vi "Material Theme Editor.vi"() -> ()   [LabVIEW 2021]
doc: "Convert existing material3 json files exported from Google to be used with TSC Material application VIs.\n\n<b>Code Developed By:</b>\nDaniel Coons\nTechnology Service Corporation\nwww.tsc.com/atcs"
uses:
  Material Theme/Material Theme.lvclass
  <vilib>/Utility/traverseref.llb/TRef TravTarget.ctl
  _theme-editor/Theme Config/Theme Config.lvclass/Theme Config.ctl
  _Material Theme SubVIs/material theme.ctl
  _Material Theme SubVIs/material json scheme.ctl
  _Material Theme SubVIs/material json palette.ctl
  Material-Scheme/Material-Scheme.lvclass/Material-Scheme.ctl
  8aff6bdd-0f42-4725-a4f4-6aecb987c99b.vi
  _theme-editor/Theme Config/Set theme path.vi
  _theme-editor/Theme Config/Set Theme Mode.vi
  Material-Scheme/data member access/get surface.vi
  Material-Scheme/data member access/Read name.vi
  _theme-editor/Theme Config/Get theme path.vi
  _theme-editor/Theme Config/Get Theme Mode.vi
  <vilib>/JDP Science/JSONtext/JSON text to Variant.vi
  _theme-editor/Theme Config/Save Configuration.vi
  Material-Scheme/View-User Colors.vi
  Material-Scheme/Material-Scheme.lvclass
  <vilib>/JDP Science/JSONtext/LVClass Serializer/JSONtext LVClass Serializer.lvclass
  Material-Palette/Material-Palette.lvclass
  user32.dll
  <vilib>/Utility/traverseref.llb/VI Scripting - Traverse.lvlib
  _theme-editor/Theme Config/Theme Config.lvclass
panel:
  in  "palette":bool
  in  "File Interaction":enum32{"convert--buton", "load--buton"}(radio)
  in  "tabs":enum32{"color", "palette", "json", "buttons"}(radio)
  in  "preview":bool
  in  "close":bool
  out "header":bool
  in  "save":bool
  in  "Theme Mode":u16(ring) items=["Light Theme", "Light Medium Contrast", "Light High Contrast", "Dark Theme", "Dark Medium Contrast", "Dark High Constrast"]
  in  "Tab Control":T1(tab)
  out "material JSON output":string
  in  "Color Level":u16(ring) items=["Primary", "Secondary", "Tertiary", "Error", "Primary Fixed", "Secondary Fixed", "Tertiary Fixed"]
  in  "Tab Control file":enum32{"convert", "load"}(tab)
  in  "json file path":path
  in  "LabVIEW material theme":path
  # "Convert a JSON M3 theme file from Google and \nuse the TSC Material Theme in a VI"
  # "Can be generated through Figma or at:   https://material-foundation.github.io/material-theme-builder/<Material Website>"
  # "Load a TSC Material Theme LabVIEW file to see modes\nand palette colors."
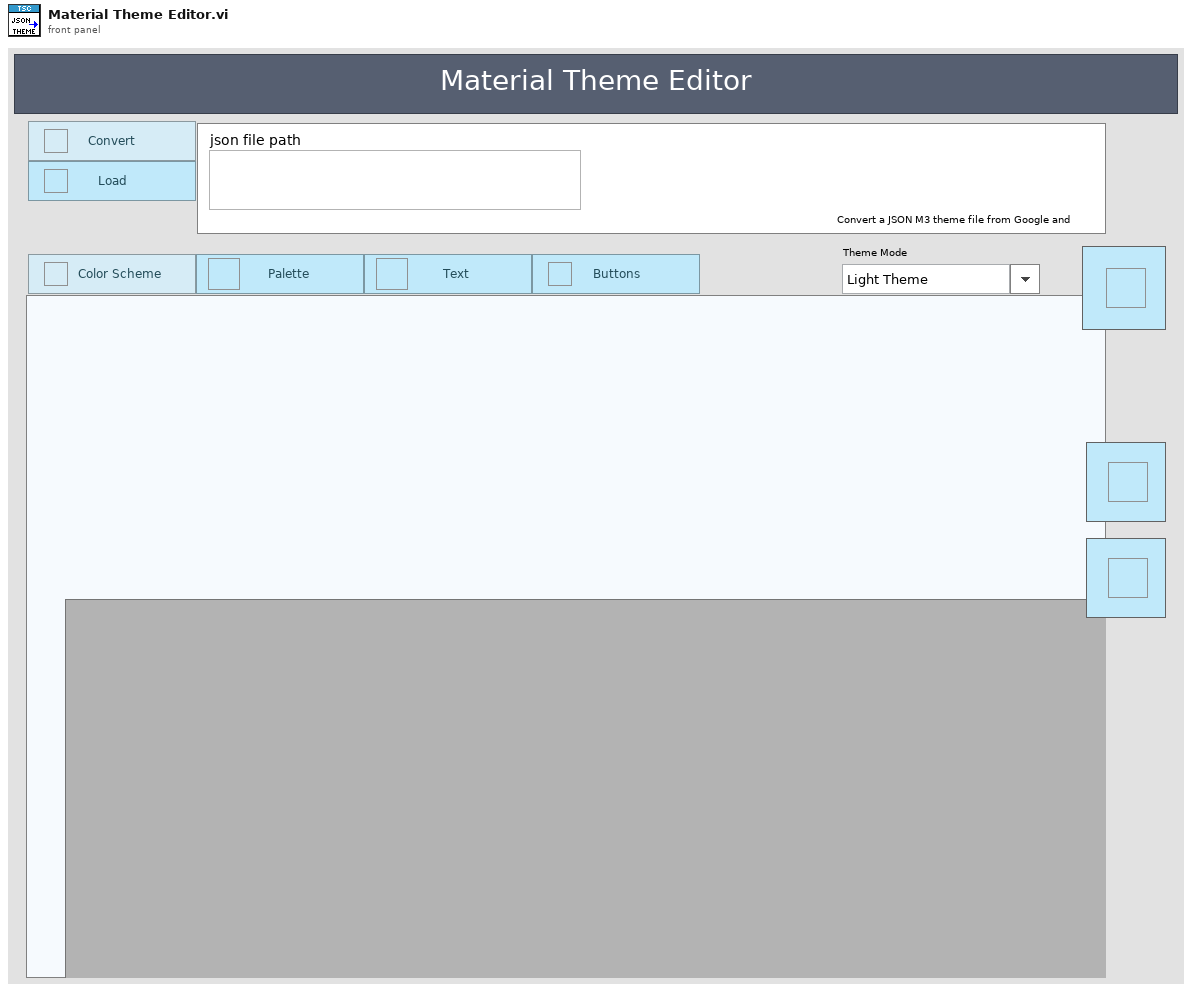
[diagram p1: front panel]
types:
  T1 = enum32{"Color Scheme", "Palette Variations", "JSON String", "buttons"}
  T2 = typedef "TRef TravTarget.ctl" = enum16{"FP", "BD", "Other"}
  T3 = typedef "material theme.ctl" = cluster{"description":string, "seed":string, "coreColors":cluster{"primary":string, "secondary":string, "tertiary":string, "error":string}, "schemes":cluster{"light":T4, "light-medium-contrast":T4, "light-high-contrast":T4, "dark":T4, "dark-medium-contrast":T4, "dark-high-contrast":T4}, "palettes":cluster{"primary":T5, "secondary":T5, "tertiary":T5, "neutral":T5, "neutral-variant":T5}}
  T4 = typedef "material json scheme.ctl" = cluster{"primary":string, "surfaceTint":string, "onPrimary":string, "primaryContainer":string, "onPrimaryContainer":string, "secondary":string, "onSecondary":string, "secondaryContainer":string, "onSecondaryContainer":string, "tertiary":string, "onTertiary":string, "tertiaryContainer":string, "onTertiaryContainer":string, "error":string, "onError":string, "errorContainer":string, "onErrorContainer":string, "background":string, "onBackground":string, "surface":string, "onSurface":string, "surfaceVariant":string, "onSurfaceVariant":string, "outline":string, "outlineVariant":string, "shadow":string, "scrim":string, "inverseSurface":string, "inverseOnSurface":string, "inversePrimary":string, "primaryFixed":string, "onPrimaryFixed":string, "primaryFixedDim":string, "onPrimaryFixedVariant":string, "secondaryFixed":string, "onSecondaryFixed":string, "secondaryFixedDim":string, "onSecondaryFixedVariant":string, "tertiaryFixed":string, "onTertiaryFixed":string, "tertiaryFixedDim":string, "onTertiaryFixedVariant":string, "surfaceDim":string, "surfaceBright":string, "surfaceContainerLowest":string, "surfaceContainerLow":string, "surfaceContainer":string, "surfaceContainerHigh":string, "surfaceContainerHighest":string}
  T5 = typedef "material json palette.ctl" = cluster{"0":string, "5":string, "10":string, "15":string, "20":string, "25":string, "30":string, "35":string, "40":string, "50":string, "60":string, "70":string, "80":string, "90":string, "95":string, "98":string, "99":string, "100":string}
  T6 = enum16{"open", "replace", "create", "open or create", "replace or create", "replace or create with confirmation"}
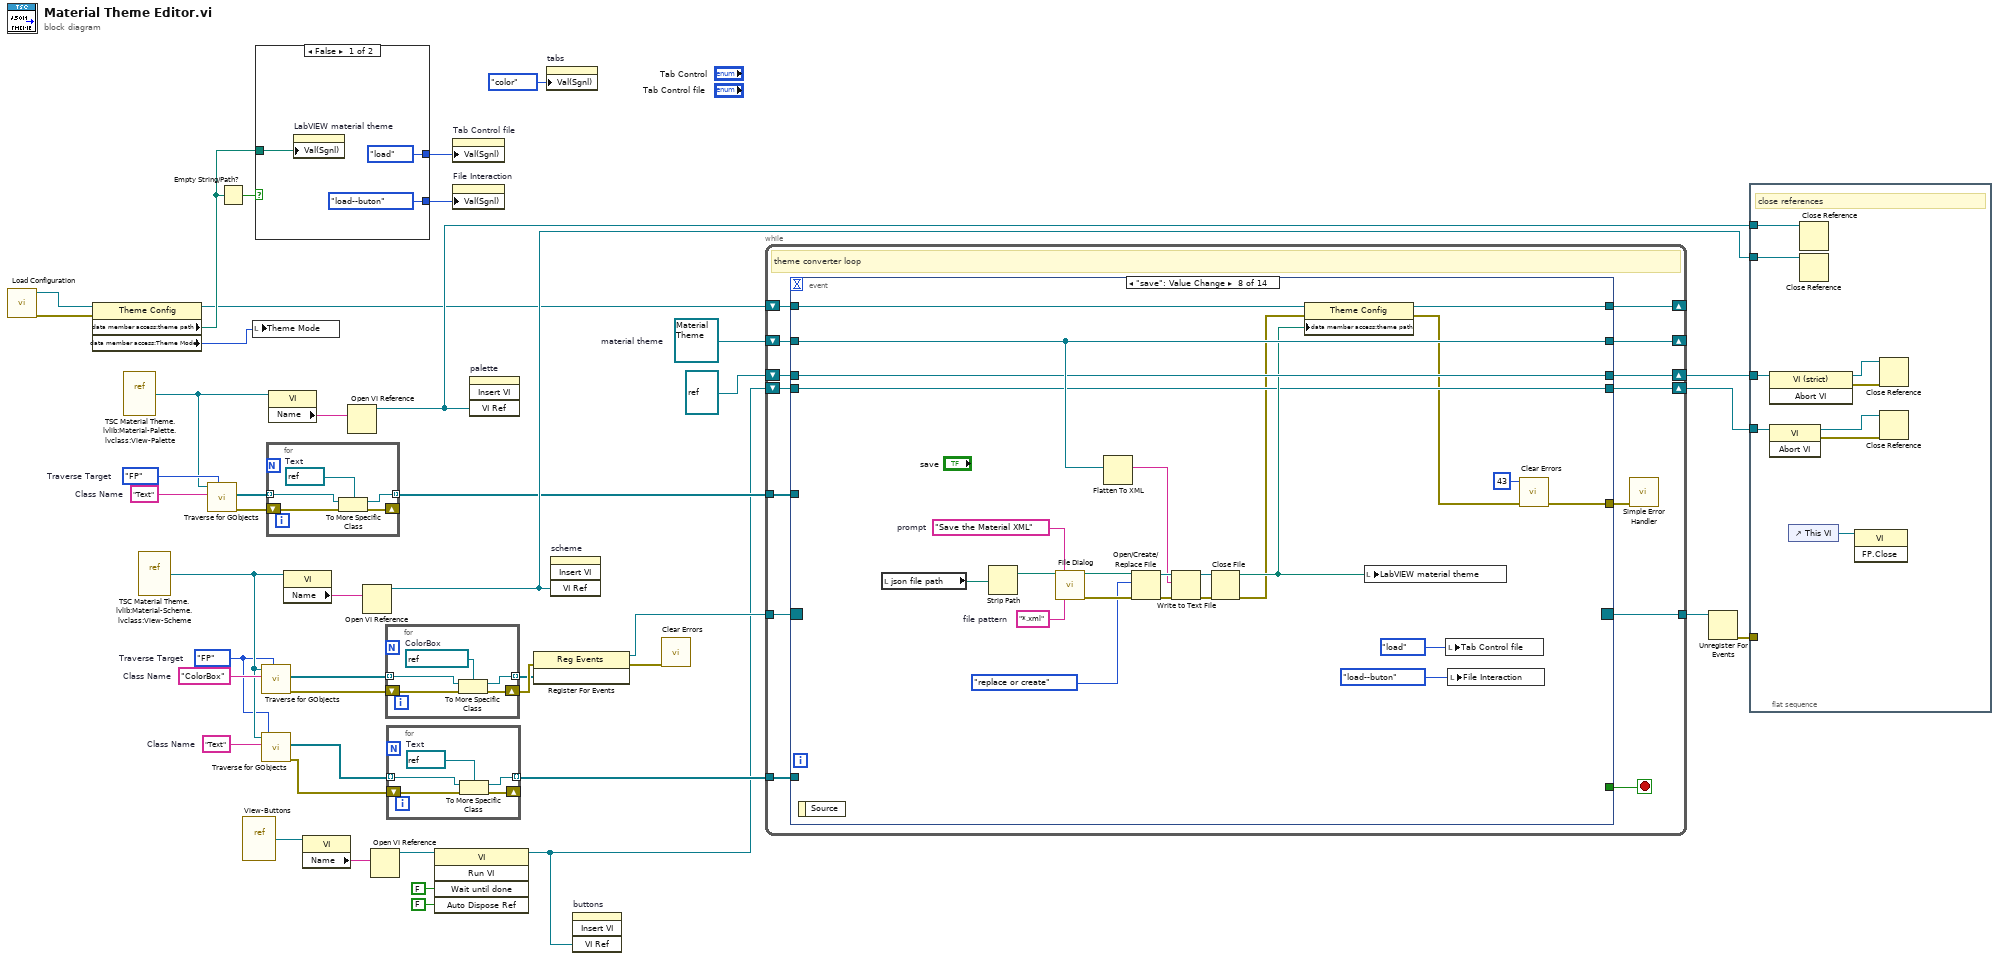
[diagram p0: block diagram]
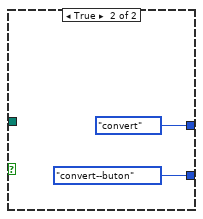
[diagram p2: hidden frame]
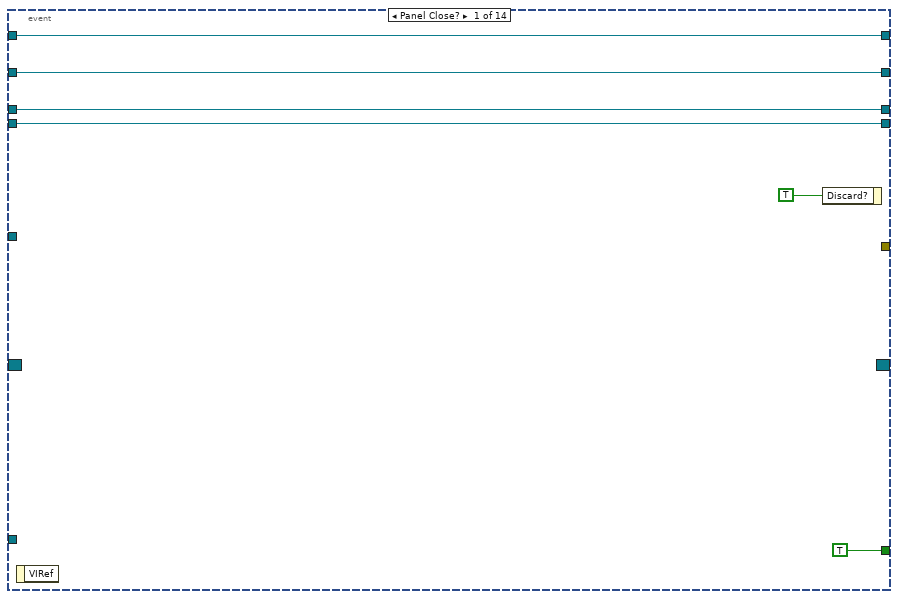
[diagram p3: hidden frame]
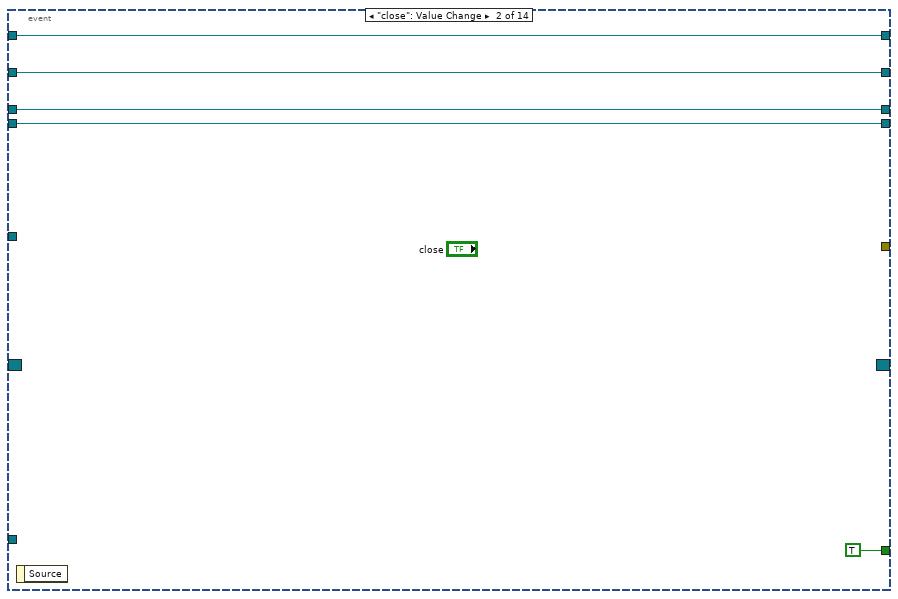
[diagram p4: hidden frame]
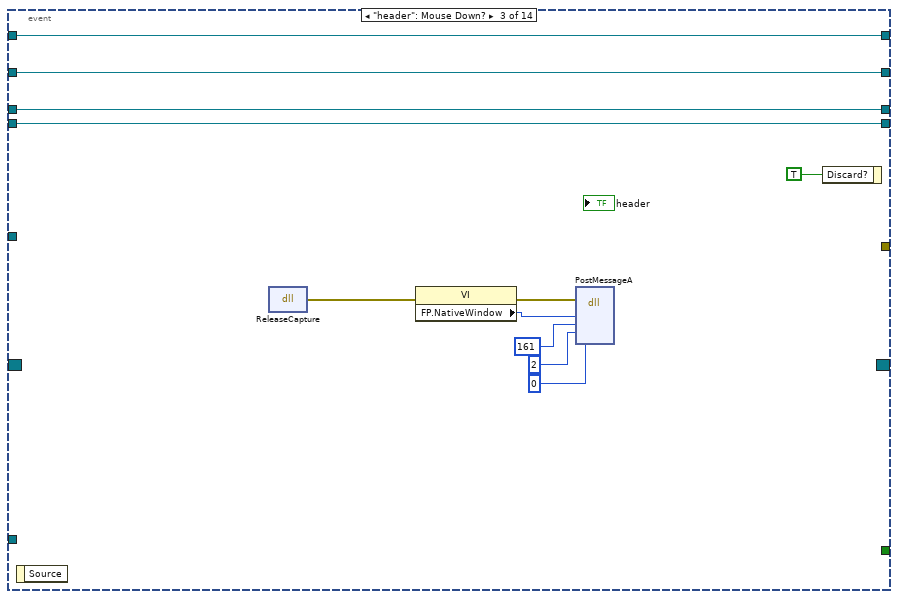
[diagram p5: hidden frame]
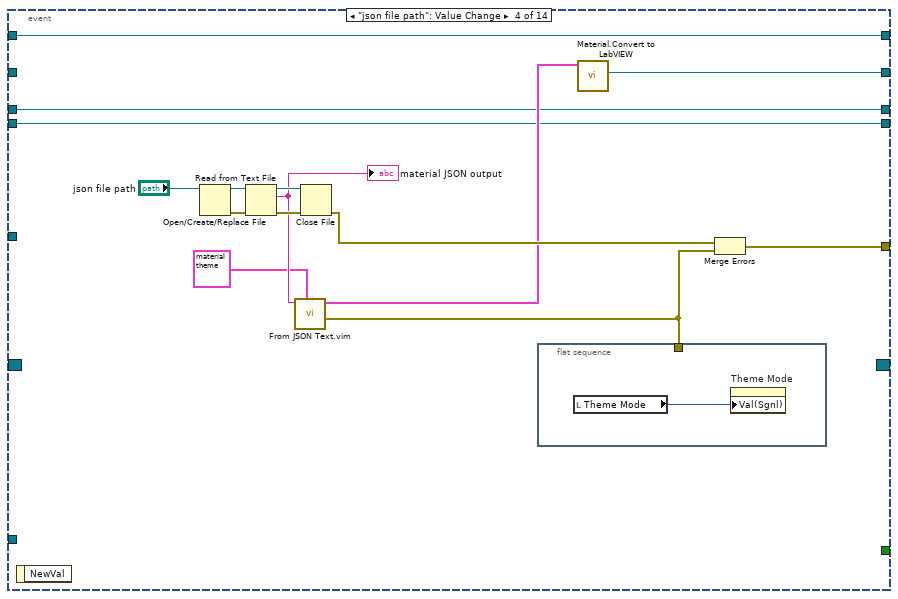
[diagram p6: hidden frame]
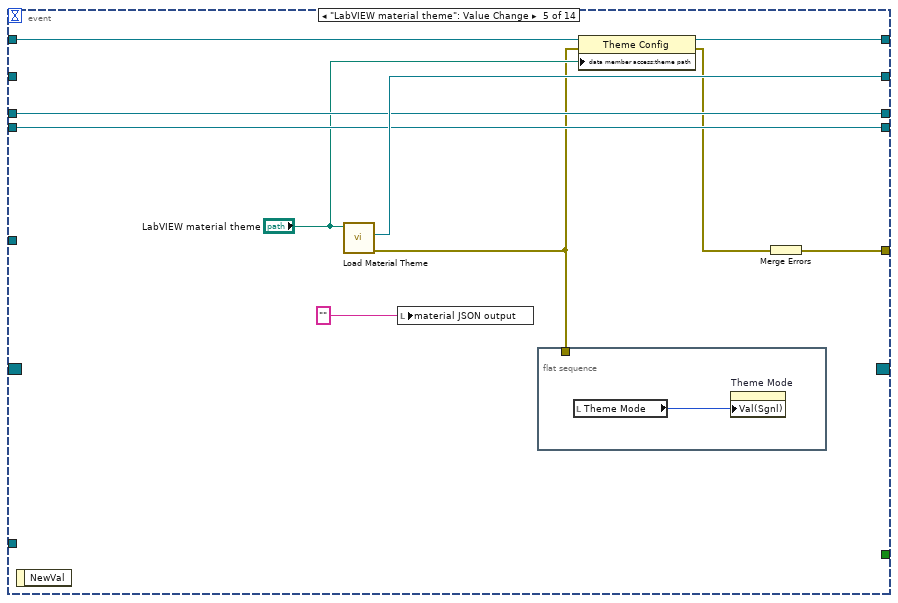
[diagram p7: hidden frame]
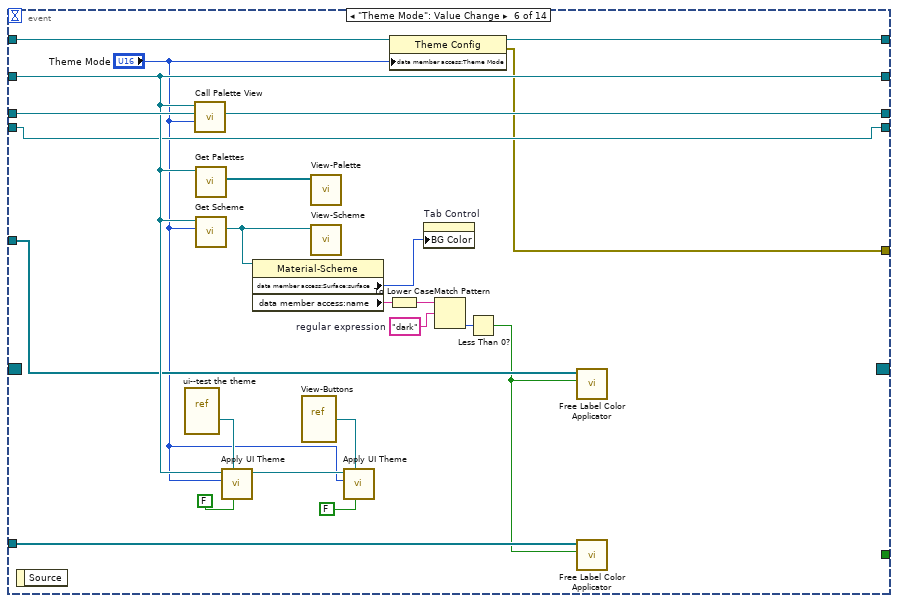
[diagram p8: hidden frame]
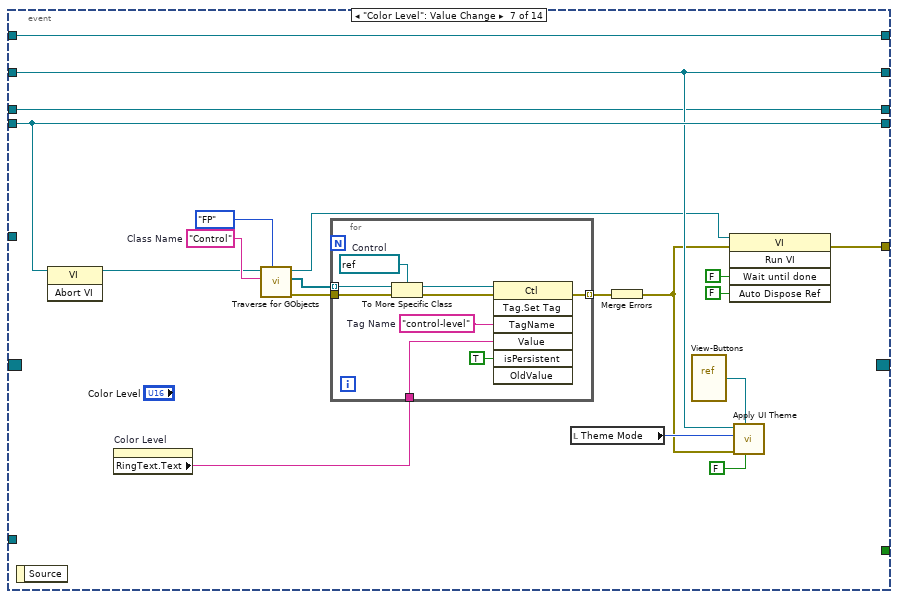
[diagram p9: hidden frame]
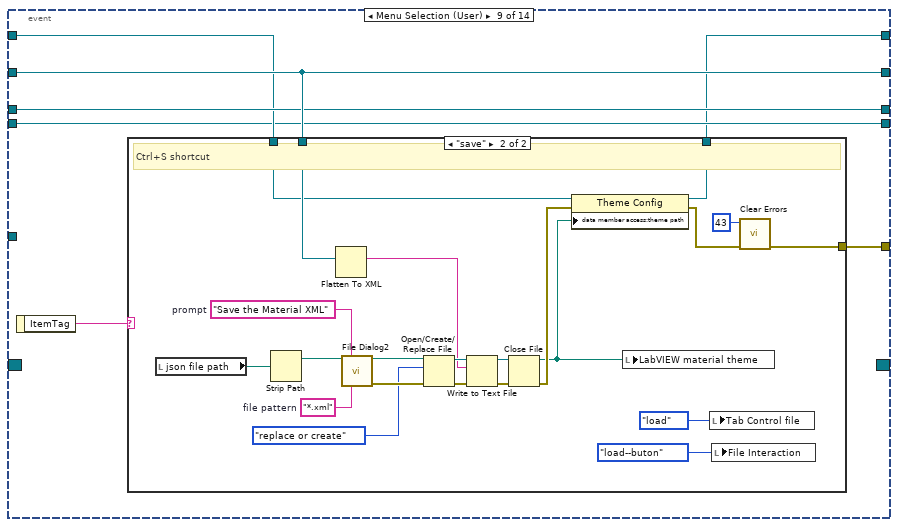
[diagram p10: hidden frame]
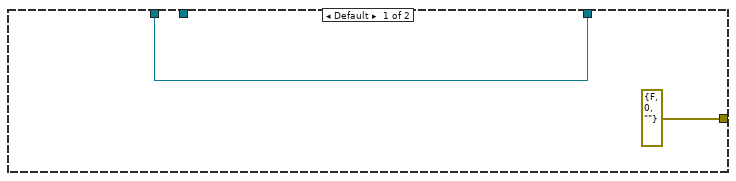
[diagram p11: hidden frame]
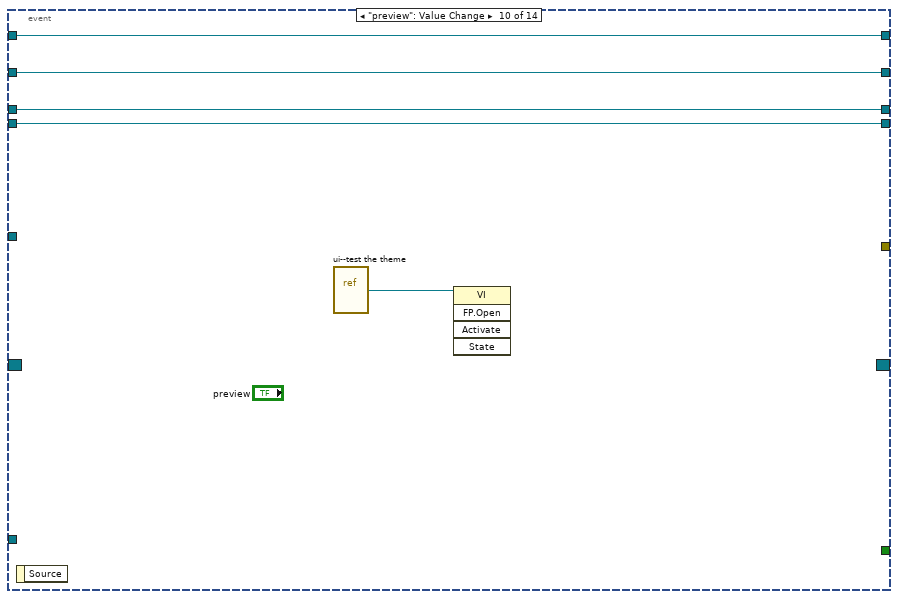
[diagram p12: hidden frame]
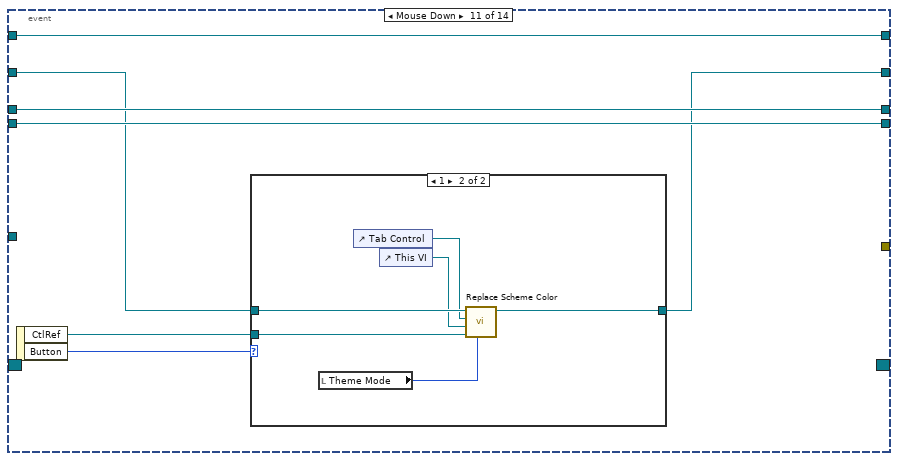
[diagram p13: hidden frame]
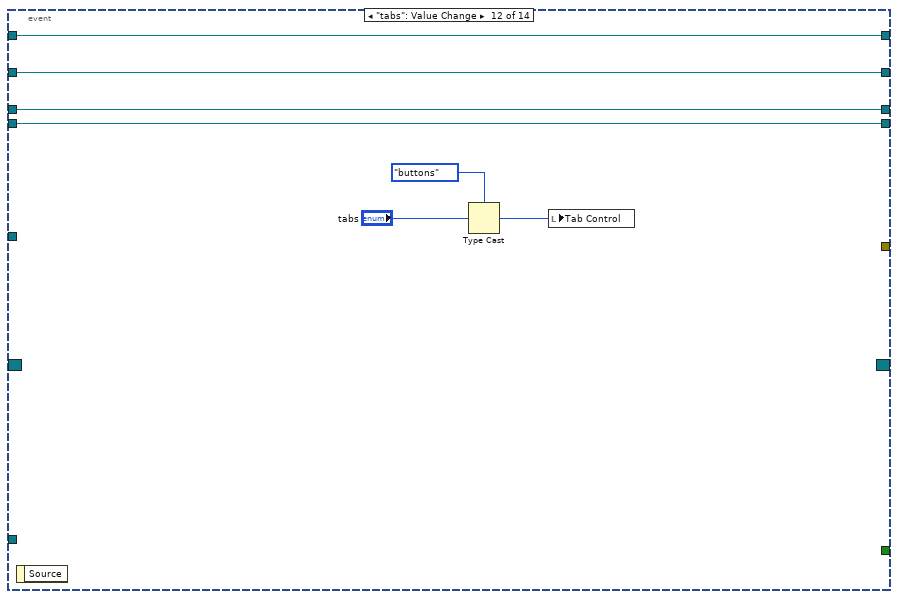
[diagram p15: hidden frame]
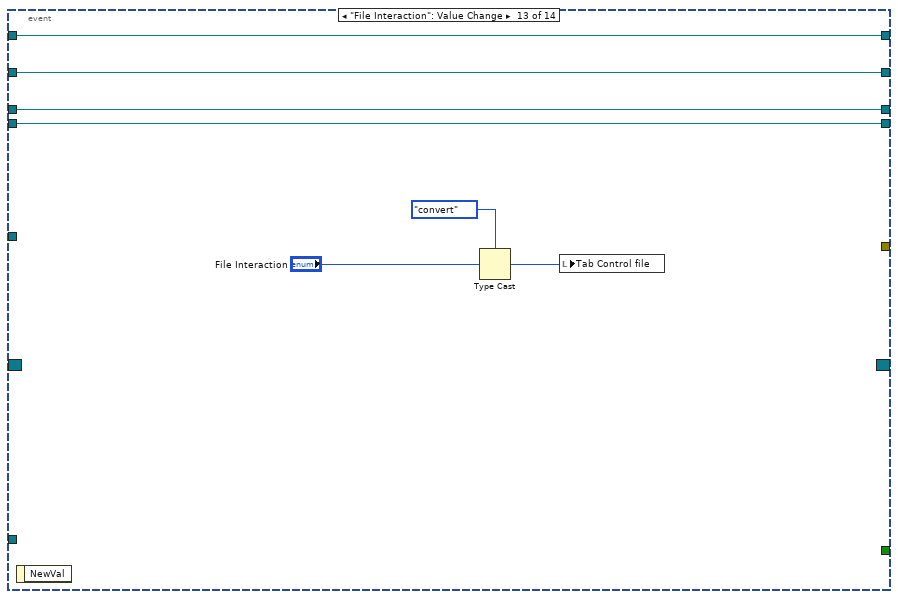
[diagram p16: hidden frame]
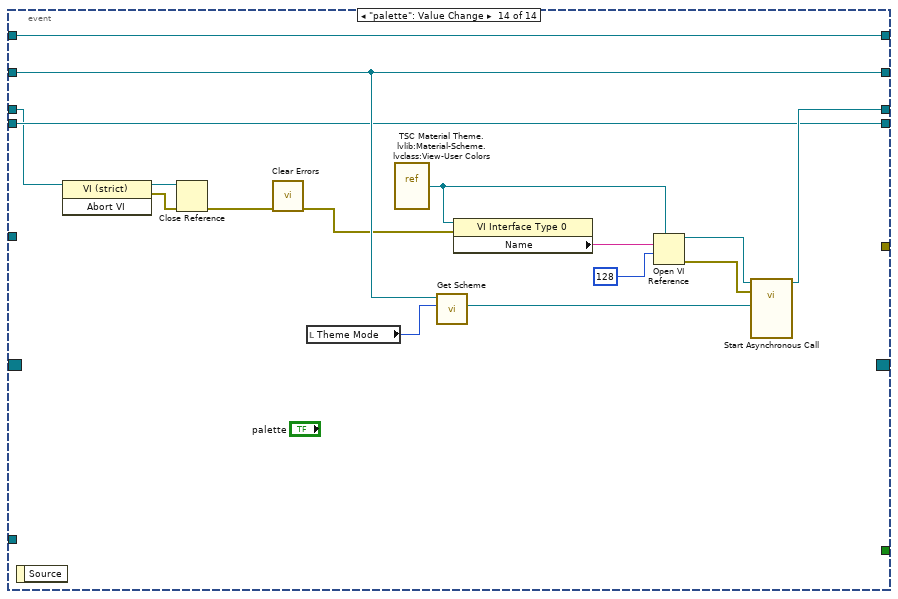
[diagram p17: hidden frame]
diagram:
  w24 = "Text"  # Class Name
  w27 = "Text"  # Class Name
  w28 = TRef_TravTarget."FP"  # Traverse Target
  w30 = refnum<class "Material Theme.lvclass"> refnum  # material theme
  w36 = "ColorBox"  # Class Name
  w22 = TRef_TravTarget."FP"  # Traverse Target
  n1 = call "Load Configuration.vi"() -> ("error out"=w10:errorcluster, "Theme Config out"=w9:refnum<class "Theme Config.lvclass">)  [unwired: 10 in]
  n2 = property class="Theme Config"(reference=w9, error in=w10) -> (reference out=w6:refnum<class "Theme Config.lvclass">, "data member access:theme path"=w8:path, "data member access:Theme Mode"=w3:u16)  [unwired: 1 out]
  n3 = vi-ref "TSC Material Theme.lvlib:Material-Palette.lvclass:View-Palette.vi"() -> (w7:refnum<vi>)
  n4 = vi-ref "TSC Material Theme.lvlib:Material-Scheme.lvclass:View-Scheme.vi"() -> (w23:refnum<vi>)
  n5 = call <vilib>:"Traverse for GObjects.vi"("Traverse Target"=w28, "Class Name"=w27, "VI Refnum"=w7) -> ("error out"=w41:errorcluster, "References"=w26:refnum<vi>[])  [unwired: 5 in, 2 out]
  n6 = Empty String/Path?(string/path=w8) -> (empty?=w29:bool)
  n7 = vi-ref "View-Buttons.vi"() -> (w17:refnum<vi>)
  n8 = local write "Theme Mode"(w3) -> ()
  n9 = case shown="False" w29 {
    tunnel: w8 -> [w47 _]
    tunnel: [enum32{"convert", "load"}."load" ("Value (Signaling)") enum32{"convert", "load"}."convert" ("Value (Signaling)")] -> w2
    tunnel: [enum32{"convert--buton", "load--buton"}."load--buton" ("Value (Signaling)") enum32{"convert--buton", "load--buton"}."convert--buton" ("Value (Signaling)")] -> w1
    frame False {
      n10 = property on="LabVIEW material theme" class="Path"("Val(Sgnl)"=w47) -> ()  [unwired: 2 in, 2 out]
    }
    frame True {
    }
  }
  n11 = call <vilib>:"Traverse for GObjects.vi"("Traverse Target"=w22, "Class Name"=w36, "VI Refnum"=w23) -> ("error out"=w44:errorcluster, "References"=w34:refnum<vi>[])  [unwired: 5 in, 2 out]
  n12 = call <vilib>:"Traverse for GObjects.vi"("Traverse Target"=w22, "Class Name"=w24, "VI Refnum"=w23) -> ("error out"=w40:errorcluster, "References"=w21:refnum<vi>[])  [unwired: 5 in, 2 out]
  n13 = for {
    tunnel: w26 -> [w51] mode=indexing
    shift-right: [w53] -> _
    shift-left: w41 -> [w54]
    tunnel: [w50] -> w25 mode=indexing
    w52 = refnum<vi> refnum  # Text
    n14 = To More Specific Class(target class=w52, reference=w51, error in=w54) -> (specific class reference=w50:refnum<vi>, error out=w53:errorcluster)
  }
  n15 = property class="VI"(reference=w7) -> ("Name"=w39:string)  [unwired: 1 in, 2 out]
  n16 = property class="VI"(reference=w23) -> ("Name"=w38:string)  [unwired: 1 in, 2 out]
  n17 = property class="VI"(reference=w17) -> ("Name"=w16:string)  [unwired: 1 in, 2 out]
  n18 = Open VI Reference(vi path=w39) -> (vi reference=w37:refnum<vi>)  [unwired: 5 in, 1 out]
  n19 = Open VI Reference(vi path=w38) -> (vi reference=w33:refnum<vi>)  [unwired: 5 in, 1 out]
  n20 = Open VI Reference(vi path=w16) -> (vi reference=w18:refnum<vi>)  [unwired: 5 in, 1 out]
  n21 = for {
    tunnel: w34 -> [w56] mode=indexing
    shift-right: [w58] -> w43
    shift-left: w44 -> [w59]
    tunnel: [w55] -> w32 mode=indexing
    w57 = refnum<vi> refnum  # ColorBox
    n22 = To More Specific Class(target class=w57, reference=w56, error in=w59) -> (specific class reference=w55:refnum<vi>, error out=w58:errorcluster)
  }
  n23 = for {
    tunnel: w21 -> [w61] mode=indexing
    shift-right: [w63] -> _
    shift-left: w40 -> [w64]
    tunnel: [w60] -> w20 mode=indexing
    w62 = refnum<vi> refnum  # Text
    n24 = To More Specific Class(target class=w62, reference=w61, error in=w64) -> (specific class reference=w60:refnum<vi>, error out=w63:errorcluster)
  }
  n25 = invoke class="VI" method="Run VI"(reference=w18, "Wait until done"=FALSE ("Wait Until Done"), "Auto Dispose Ref"=FALSE ("Auto Dispose Reference")) -> (reference out=w13:refnum<vi>)  [unwired: 2 in, 4 out]
  n26 = property on="Tab Control file" class="TabCtl (strict)"("Val(Sgnl)"=w2) -> ()  [unwired: 2 in, 2 out]
  n27 = property on="File Interaction" class="RadioBtnsControl (strict)"("Val(Sgnl)"=w1) -> ()  [unwired: 2 in, 2 out]
  n28 = invoke on="palette" class="SubPnl" method="Insert VI"("VI Ref"=w37) -> ()  [unwired: 3 in, 4 out]
  n29 = register-events(error in=w43, w32) -> (reference out=w35:refnum<event-registration>, error out=w42:errorcluster)  [unwired: 1 in]
  n30 = property on="tabs" class="RadioBtnsControl (strict)"("Val(Sgnl)"=enum32{"color", "palette", "json", "buttons"}."color" ("Value (Signaling)")) -> ()  [unwired: 2 in, 2 out]
  n31 = invoke on="scheme" class="SubPnl" method="Insert VI"("VI Ref"=w33) -> ()  [unwired: 3 in, 4 out]
  n32 = invoke on="buttons" class="SubPnl" method="Insert VI"("VI Ref"=w13) -> ()  [unwired: 3 in, 4 out]
  n33 = call <vilib>:"Clear Errors.vi"("error in (no error)"=w42) -> ()  [unwired: 5 in, 2 out]
  n34 = while {
    shift-right: [w76] -> _
    shift-left: w30 -> [w75]
    tunnel: w35 -> [w74]
    tunnel: [w73] -> w31
    tunnel: w25 -> [w72]
    tunnel: w20 -> [w71]
    shift-right: [w69] -> w12
    shift-left: refnum<vi> refnum -> [w68]
    shift-right: [w66] -> _
    shift-left: w6 -> [w67]
    shift-right: [w65] -> w4
    shift-left: w13 -> [w70]
    stop <- w77 stop-if-true
    # "theme converter loop"
    n35 = event shown="[7] \"save\": Value Change" {
      selector: w74 -> [_ _ _ _ _ _ _ _ _ _ _ _ _ _]
      dyn-events: [_ _ _ _ _ _ _ _ _ _ _ _ _ _] -> w73
      timeout: _ -> [_ _ _ _ _ _ _ _ _ _ _ _ _ _]
      tunnel: [TRUE TRUE _ _ _ _ _ _ _ _ _ _ _ _] -> w77
      tunnel: [w82 w89 w93 w108 w125 w137 w156 w196 w208 w238 w239 w259 w263 w282] -> w76
      tunnel: w75 -> [w82 w89 w93 _ _ w137 w156 w196 w208 w238 w240 w259 w263 w282]
      tunnel: [_ _ _ w112 w126 w128 w162 w179 w209 _ _ _ _ _] -> w78
      tunnel: w72 -> [_ _ _ _ _ w132 _ _ _ _ _ _ _ _]
      tunnel: w71 -> [_ _ _ _ _ w141 _ _ _ _ _ _ _ _]
      tunnel: w70 -> [w79 w85 w90 w101 w121 w133 w167 w182 w204 w234 w242 w253 w260 w272]
      tunnel: [w81 w87 w92 w103 w123 w136 w152 w188 w206 w236 w244 w255 w262 w274] -> w69
      tunnel: w68 -> [w81 w87 w92 w103 w123 w138 w152 w188 w206 w236 w244 w255 w262 w269]
      tunnel: w67 -> [w80 w86 w91 w102 w122 w134 w151 w185 w205 w235 w243 w254 w261 w273]
      tunnel: [w80 w86 w91 w102 w120 w130 w151 w184 w203 w235 w243 w254 w261 w273] -> w66
      tunnel: [w79 w85 w90 w101 w121 w133 w167 w182 w204 w234 w242 w253 w260 w272] -> w65
      event Panel Close? {
        n36 = event-data() -> ()  [unwired: 1 in, 1 out]
        n37 = event-data("Discard?"=TRUE) -> ()  [unwired: 1 in, 1 out]
      }
      event "close": Value Change {
        n38 = event-data() -> ()  [unwired: 1 in, 1 out]
      }
      event "header": Mouse Down? {
        n39 = event-data() -> ()  [unwired: 1 in, 1 out]
        n40 = dll-call lib="user32.dll" fn="ReleaseCapture"() -> (error out=w100:errorcluster)  [unwired: 4 in, 1 out]
        n41 = property class="VI"(error in=w100) -> (error out=w99:errorcluster, "FP.NativeWindow"=w94:u64)  [unwired: 1 in, 1 out]
        n42 = dll-call lib="user32.dll" fn="PostMessageA"(error in=w99, "hWnd"=w94, "Msg"=161, "wParam"=2, "lParam"=0) -> ()  [unwired: 7 in, 2 out]
        n43 = event-data("Discard?"=TRUE) -> ()  [unwired: 1 in, 1 out]
      }
      event "json file path": Value Change {
        n44 = event-data() -> ()  [unwired: 1 in, 1 out]
        n45 = Open/Create/Replace File(file path (use dialog)="json file path") -> (refnum out=w109:refnum<file>, error out=w114:errorcluster)  [unwired: 5 in, 1 out]
        n46 = Read from Text File(file (use dialog)=w109, error in=w114) -> (refnum out=w110:refnum<file>, text=w107:string, error out=w115:errorcluster)  [unwired: 2 in, 1 out]
        "material JSON output" <- w107
        n47 = call "From JSON Text.vim"("Data Type and Default Value"=T3 {"description"="", "seed"="", "coreColors"={"primary"="", "secondary"="", "tertiary"="", "error"=""}, "schemes"={"light"={"primary"="", "surfaceTint"="", "onPrimary"="", "primaryContainer"="0", "onPrimaryContainer"="0", "secondary"="0", "onSecondary"="0", "secondaryContainer"="0", "onSecondaryContainer"="0", "tertiary"="0", "onTertiary"="0", "tertiaryContainer"="0", "onTertiaryContainer"="0", "error"="0", "onError"="0", "errorContainer"="0", "onErrorContainer"="0", "background"="0", "onBackground"="0", "surface"="0", "onSurface"="0", "surfaceVariant"="0", "onSurfaceVariant"="0", "outline"="0", "outlineVariant"="0", "shadow"="0", "scrim"="0", "inverseSurface"="0", "inverseOnSurface"="0", "inversePrimary"="", "primaryFixed"="0", "onPrimaryFixed"="0", "primaryFixedDim"="0", "onPrimaryFixedVariant"="0", "secondaryFixed"="0", "onSecondaryFixed"="0", "secondaryFixedDim"="0", "onSecondaryFixedVariant"="0", "tertiaryFixed"="0", "onTertiaryFixed"="0", "tertiaryFixedDim"="0", "onTertiaryFixedVariant"="0", "surfaceDim"="0", "surfaceBright"="0", "surfaceContainerLowest"="0", "surfaceContainerLow"="0", "surfaceContainer"="0", "surfaceContainerHigh"="0", "surfaceContainerHighest"="0"}, "light-medium-contrast"={"primary"="", "surfaceTint"="", "onPrimary"="", "primaryContainer"="0", "onPrimaryContainer"="0", "secondary"="0", "onSecondary"="0", "secondaryContainer"="0", "onSecondaryContainer"="0", "tertiary"="0", "onTertiary"="0", "tertiaryContainer"="0", "onTertiaryContainer"="0", "error"="0", "onError"="0", "errorContainer"="0", "onErrorContainer"="0", "background"="0", "onBackground"="0", "surface"="0", "onSurface"="0", "surfaceVariant"="0", "onSurfaceVariant"="0", "outline"="0", "outlineVariant"="0", "shadow"="0", "scrim"="0", "inverseSurface"="0", "inverseOnSurface"="0", "inversePrimary"="", "primaryFixed"="0", "onPrimaryFixed"="0", "primaryFixedDim"="0", "onPrimaryFixedVariant"="0", "secondaryFixed"="0", "onSecondaryFixed"="0", "secondaryFixedDim"="0", "onSecondaryFixedVariant"="0", "tertiaryFixed"="0", "onTertiaryFixed"="0", "tertiaryFixedDim"="0", "onTertiaryFixedVariant"="0", "surfaceDim"="0", "surfaceBright"="0", "surfaceContainerLowest"="0", "surfaceContainerLow"="0", "surfaceContainer"="0", "surfaceContainerHigh"="0", "surfaceContainerHighest"="0"}, "light-high-contrast"={"primary"="", "surfaceTint"="", "onPrimary"="", "primaryContainer"="0", "onPrimaryContainer"="0", "secondary"="0", "onSecondary"="0", "secondaryContainer"="0", "onSecondaryContainer"="0", "tertiary"="0", "onTertiary"="0", "tertiaryContainer"="0", "onTertiaryContainer"="0", "error"="0", "onError"="0", "errorContainer"="0", "onErrorContainer"="0", "background"="0", "onBackground"="0", "surface"="0", "onSurface"="0", "surfaceVariant"="0", "onSurfaceVariant"="0", "outline"="0", "outlineVariant"="0", "shadow"="0", "scrim"="0", "inverseSurface"="0", "inverseOnSurface"="0", "inversePrimary"="", "primaryFixed"="0", "onPrimaryFixed"="0", "primaryFixedDim"="0", "onPrimaryFixedVariant"="0", "secondaryFixed"="0", "onSecondaryFixed"="0", "secondaryFixedDim"="0", "onSecondaryFixedVariant"="0", "tertiaryFixed"="0", "onTertiaryFixed"="0", "tertiaryFixedDim"="0", "onTertiaryFixedVariant"="0", "surfaceDim"="0", "surfaceBright"="0", "surfaceContainerLowest"="0", "surfaceContainerLow"="0", "surfaceContainer"="0", "surfaceContainerHigh"="0", "surfaceContainerHighest"="0"}, "dark"={"primary"="", "surfaceTint"="", "onPrimary"="", "primaryContainer"="0", "onPrimaryContainer"="0", "secondary"="0", "onSecondary"="0", "secondaryContainer"="0", "onSecondaryContainer"="0", "tertiary"="0", "onTertiary"="0", "tertiaryContainer"="0", "onTertiaryContainer"="0", "error"="0", "onError"="0", "errorContainer"="0", "onErrorContainer"="0", "background"="0", "onBackground"="0", "surface"="0", "onSurface"="0", "surfaceVariant"="0", "onSurfaceVariant"="0", "outline"="0", "outlineVariant"="0", "shadow"="0", "scrim"="0", "inverseSurface"="0", "inverseOnSurface"="0", "inversePrimary"="", "primaryFixed"="0", "onPrimaryFixed"="0", "primaryFixedDim"="0", "onPrimaryFixedVariant"="0", "secondaryFixed"="0", "onSecondaryFixed"="0", "secondaryFixedDim"="0", "onSecondaryFixedVariant"="0", "tertiaryFixed"="0", "onTertiaryFixed"="0", "tertiaryFixedDim"="0", "onTertiaryFixedVariant"="0", "surfaceDim"="0", "surfaceBright"="0", "surfaceContainerLowest"="0", "surfaceContainerLow"="0", "surfaceContainer"="0", "surfaceContainerHigh"="0", "surfaceContainerHighest"="0"}, "dark-medium-contrast"={"primary"="", "surfaceTint"="", "onPrimary"="", "primaryContainer"="0", "onPrimaryContainer"="0", "secondary"="0", "onSecondary"="0", "secondaryContainer"="0", "onSecondaryContainer"="0", "tertiary"="0", "onTertiary"="0", "tertiaryContainer"="0", "onTertiaryContainer"="0", "error"="0", "onError"="0", "errorContainer"="0", "onErrorContainer"="0", "background"="0", "onBackground"="0", "surface"="0", "onSurface"="0", "surfaceVariant"="0", "onSurfaceVariant"="0", "outline"="0", "outlineVariant"="0", "shadow"="0", "scrim"="0", "inverseSurface"="0", "inverseOnSurface"="0", "inversePrimary"="", "primaryFixed"="0", "onPrimaryFixed"="0", "primaryFixedDim"="0", "onPrimaryFixedVariant"="0", "secondaryFixed"="0", "onSecondaryFixed"="0", "secondaryFixedDim"="0", "onSecondaryFixedVariant"="0", "tertiaryFixed"="0", "onTertiaryFixed"="0", "tertiaryFixedDim"="0", "onTertiaryFixedVariant"="0", "surfaceDim"="0", "surfaceBright"="0", "surfaceContainerLowest"="0", "surfaceContainerLow"="0", "surfaceContainer"="0", "surfaceContainerHigh"="0", "surfaceContainerHighest"="0"}, "dark-high-contrast"={"primary"="", "surfaceTint"="", "onPrimary"="", "primaryContainer"="0", "onPrimaryContainer"="0", "secondary"="0", "onSecondary"="0", "secondaryContainer"="0", "onSecondaryContainer"="0", "tertiary"="0", "onTertiary"="0", "tertiaryContainer"="0", "onTertiaryContainer"="0", "error"="0", "onError"="0", "errorContainer"="0", "onErrorContainer"="0", "background"="0", "onBackground"="0", "surface"="0", "onSurface"="0", "surfaceVariant"="0", "onSurfaceVariant"="0", "outline"="0", "outlineVariant"="0", "shadow"="0", "scrim"="0", "inverseSurface"="0", "inverseOnSurface"="0", "inversePrimary"="", "primaryFixed"="0", "onPrimaryFixed"="0", "primaryFixedDim"="0", "onPrimaryFixedVariant"="0", "secondaryFixed"="0", "onSecondaryFixed"="0", "secondaryFixedDim"="0", "onSecondaryFixedVariant"="0", "tertiaryFixed"="0", "onTertiaryFixed"="0", "tertiaryFixedDim"="0", "onTertiaryFixedVariant"="0", "surfaceDim"="0", "surfaceBright"="0", "surfaceContainerLowest"="0", "surfaceContainerLow"="0", "surfaceContainer"="0", "surfaceContainerHigh"="0", "surfaceContainerHighest"="0"}}, "palettes"={"primary"={"0"="0", "5"="0", "10"="0", "15"="0", "20"="0", "25"="0", "30"="0", "35"="0", "40"="0", "50"="0", "60"="0", "70"="0", "80"="0", "90"="0", "95"="0", "98"="0", "99"="0", "100"="0"}, "secondary"={"0"="0", "5"="0", "10"="0", "15"="0", "20"="0", "25"="0", "30"="0", "35"="0", "40"="0", "50"="0", "60"="0", "70"="0", "80"="0", "90"="0", "95"="0", "98"="0", "99"="0", "100"="0"}, "tertiary"={"0"="0", "5"="0", "10"="0", "15"="0", "20"="0", "25"="0", "30"="0", "35"="0", "40"="0", "50"="0", "60"="0", "70"="0", "80"="0", "90"="0", "95"="0", "98"="0", "99"="0", "100"="0"}, "neutral"={"0"="0", "5"="0", "10"="0", "15"="0", "20"="0", "25"="0", "30"="0", "35"="0", "40"="0", "50"="0", "60"="0", "70"="0", "80"="0", "90"="0", "95"="0", "98"="0", "99"="0", "100"="0"}, "neutral-variant"={"0"="0", "5"="0", "10"="0", "15"="0", "20"="0", "25"="0", "30"="0", "35"="0", "40"="0", "50"="0", "60"="0", "70"="0", "80"="0", "90"="0", "95"="0", "98"="0", "99"="0", "100"="0"}}}, "JSON"=w107) -> ("error out"=w111:errorcluster, "Data out"=w105:T3)  [unwired: 8 in]
        n48 = Close File(refnum=w110, error in=w115) -> (error out=w113:errorcluster)  [unwired: 1 out]
        n49 = flat-sequence {
          tunnel: w111 -> [_]
          frame #0 {
            n50 = local read "Theme Mode"() -> (w116:u16)
            n51 = property on="Theme Mode" class="Ring (strict)"("Val(Sgnl)"=w116) -> ()  [unwired: 2 in, 2 out]
          }
        }
        n52 = call "Material.Convert to LabVIEW.vi"("material.json string"=w105) -> ("output cluster"=w108:refnum<class "Material Theme.lvclass">)  [unwired: 10 in]
        n53 = Merge Errors(w113, w111) -> (w112:errorcluster)
      }
      event "LabVIEW material theme": Value Change {
        n54 = event-data() -> ()  [unwired: 1 in, 1 out]
        n55 = call "Load Material Theme.vi"("file path (use dialog)"="LabVIEW material theme") -> ("error out"=w118:errorcluster, "Theme"=w125:refnum<class "Material Theme.lvclass">)  [unwired: 9 in]
        n56 = local write "material JSON output"("") -> ()
        n57 = flat-sequence {
          tunnel: w118 -> [_]
          frame #0 {
            n58 = local read "Theme Mode"() -> (w127:u16)
            n59 = property on="Theme Mode" class="Ring (strict)"("Val(Sgnl)"=w127) -> ()  [unwired: 2 in, 2 out]
          }
        }
        n60 = property class="Theme Config"(reference=w122, error in=w118, "data member access:theme path"="LabVIEW material theme") -> (reference out=w120:refnum<class "Theme Config.lvclass">, error out=w117:errorcluster)
        n61 = Merge Errors(w117) -> (w126:errorcluster)
      }
      event "Theme Mode": Value Change {
        w144 = "dark"  # regular expression
        n62 = event-data() -> ()  [unwired: 1 in, 1 out]
        n63 = vi-ref "ui--test the theme.vi"() -> (w149:refnum<vi>)
        n64 = call "Call Palette View.vi"("Theme Mode"="Theme Mode", "VI ref in"=w138, "Material Theme"=w137) -> ("VI ref"=w136:refnum<vi>)  [unwired: 7 in, 1 out]
        n65 = call "Get Palettes.vi"("Material Theme in"=w137) -> ("Material-Scheme"=w150:refnum<class "Material-Palette.lvclass">[])  [unwired: 8 in, 2 out]
        n66 = call "Get Scheme.vi"("Theme"="Theme Mode", "Material Theme in"=w137) -> ("Material-Scheme"=w147:refnum<class "Material-Scheme.lvclass">)  [unwired: 7 in, 2 out]
        n67 = call "Apply UI Theme.vi"("save?"=FALSE, "VI Refnum"=w149, "Theme Mode"="Theme Mode", "Material Theme in"=w137) -> ("Material Theme out"=w135:refnum<class "Material Theme.lvclass">)  [unwired: 6 in, 1 out]
        n68 = property class="Material-Scheme"(reference=w147) -> ("data member access:Surface:surface"=w146:u32, "data member access:name"=w145:string)  [unwired: 1 in, 2 out]
        n69 = vi-ref "View-Buttons.vi"() -> (w139:refnum<vi>)
        n70 = call "View-Palette.vi"("Array"=w150) -> ()  [unwired: 11 in]
        n71 = call "View-Scheme.vi"("Material-Scheme.lvclass"=w147) -> ()  [unwired: 11 in]
        n72 = call "Apply UI Theme.vi"("save?"=FALSE, "VI Refnum"=w139, "Theme Mode"="Theme Mode", "Material Theme in"=w135) -> ()  [unwired: 6 in, 2 out]
        n73 = To Lower Case(string=w145) -> (all lower case string=w143:string)
        n74 = property class="Theme Config"(reference=w134, "data member access:Theme Mode"="Theme Mode") -> (reference out=w130:refnum<class "Theme Config.lvclass">, error out=w128:errorcluster)  [unwired: 1 in]
        n75 = property on="Tab Control" class="TabCtl (strict)"("BG Color"=w146) -> ()  [unwired: 2 in, 2 out]
        n76 = Match Pattern(string=w143, regular expression=w144) -> (offset past match=w142:i32)  [unwired: 1 in, 3 out]
        n77 = Less Than 0?(x=w142) -> (x < 0?=w131:bool)
        n78 = call "Free Label Color Applicator.vi"("Dark Text?"=w131, "Text Labels"=w132) -> ()  [unwired: 10 in]
        n79 = call "Free Label Color Applicator.vi"("Dark Text?"=w131, "Text Labels"=w141) -> ()  [unwired: 10 in]
      }
      event "Color Level": Value Change {
        w169 = "Control"  # Class Name
        n80 = event-data() -> ()  [unwired: 1 in, 1 out]
        n81 = invoke class="VI" method="Abort VI"(reference=w167) -> (reference out=w161:refnum<vi>)  [unwired: 2 in, 2 out]
        n82 = property on="Color Level" class="Ring (strict)"() -> ("RingText.Text"=w164:string)  [unwired: 2 in, 2 out]
        n83 = call <vilib>:"Traverse for GObjects.vi"("Traverse Target"=TRef_TravTarget."FP", "Class Name"=w169, "VI Refnum"=w161) -> ("error out"=w165:errorcluster, "References"=w166:refnum<vi>[], "dup VI Refnum"=w153:refnum<vi>)  [unwired: 5 in, 1 out]
        n84 = for {
          tunnel: w166 -> [w177] mode=indexing
          tunnel: w165 -> [w176]
          tunnel: w164 -> [w172]
          tunnel: [w170] -> w163 mode=indexing
          w175 = refnum<vi> refnum  # Control
          w178 = "control-level"  # Tag Name
          n85 = To More Specific Class(target class=w175, reference=w177, error in=w176) -> (specific class reference=w173:refnum<vi>, error out=w174:errorcluster)
          n86 = invoke class="Ctl" method="Tag.Set Tag"(reference=w173, error in=w174, "TagName"=w178, "Value"=w172, "isPersistent"=TRUE ("Is Persistent?")) -> (error out=w170:errorcluster)  [unwired: 2 in, 6 out]
        }
        n87 = local read "Theme Mode"() -> (w155:u16)
        n88 = Merge Errors(w163) -> (w154:errorcluster)
        n89 = vi-ref "View-Buttons.vi"() -> (w158:refnum<vi>)
        n90 = invoke class="VI" method="Run VI"(reference=w153, error in=w154, "Wait until done"=FALSE ("Wait Until Done"), "Auto Dispose Ref"=FALSE ("Auto Dispose Reference")) -> (error out=w162:errorcluster)  [unwired: 1 in, 4 out]
        n91 = call "Apply UI Theme.vi"("save?"=FALSE, "VI Refnum"=w158, "error in (no error)"=w154, "Theme Mode"=w155, "Material Theme in"=w156) -> ()  [unwired: 5 in, 2 out]
      }
      event "save": Value Change {
        w189 = "Save the Material XML"  # prompt
        w192 = "*.xml"  # file pattern
        n92 = event-data() -> ()  [unwired: 1 in, 1 out]
        n93 = local read "json file path"() -> (w191:path)
        n94 = Strip Path(path=w191) -> (stripped path=w190:path)  [unwired: 1 out]
        n95 = call "File Dialog"("start path"=w190, "prompt"=w189, "pattern (all files)"=w192) -> ("selected path"=w193:path, "error out"=w200:errorcluster)  [unwired: 9 in, 2 out]
        n96 = Flatten To XML(6:w196) -> (2:w195:string)
        n97 = Open/Create/Replace File(file path (use dialog)=w193, error in=w200, operation (0:open)=T6."replace or create") -> (refnum out=w198:refnum<file>, error out=w201:errorcluster)  [unwired: 3 in, 1 out]
        n98 = Write to Text File(file (use dialog)=w198, text=w195, error in=w201) -> (refnum out=w197:refnum<file>, error out=w202:errorcluster)  [unwired: 1 in, 1 out]
        n99 = Close File(refnum=w197, error in=w202) -> (path=w183:path, error out=w181:errorcluster)
        n100 = property class="Theme Config"(reference=w185, error in=w181, "data member access:theme path"=w183) -> (reference out=w184:refnum<class "Theme Config.lvclass">, error out=w180:errorcluster)
        n101 = local write "LabVIEW material theme"(w183) -> ()
        n102 = local write "Tab Control file"(enum32{"convert", "load"}."load" ("Tab Control file")) -> ()
        n103 = local write "File Interaction"(enum32{"convert--buton", "load--buton"}."load--buton" ("File Interaction")) -> ()
        n104 = call <vilib>:"Clear Errors.vi"("error in (no error)"=w180, "specific error code to clear (0: all)"=43) -> ("error out"=w179:errorcluster)  [unwired: 4 in, 1 out]
      }
      event Menu Selection (User) {
        n105 = event-data() -> ("ItemTag"=w207:string)  [unwired: 1 in]
        n106 = case shown="\"save\"" w207 {
          tunnel: w208 -> [_ w230]
          tunnel: [errorcluster {"status"=FALSE, "code"=0, "source"=""} ("error out") w212] -> w209
          tunnel: w205 -> [w210 w217]
          tunnel: [w210 w216] -> w203
          frame Default {
          }
          frame "save" {
            w223 = "Save the Material XML"  # prompt
            w222 = "*.xml"  # file pattern
            # "Ctrl+S shortcut"
            n107 = local read "json file path"() -> (w225:path)
            n108 = Strip Path(path=w225) -> (stripped path=w224:path)  [unwired: 1 out]
            n109 = Flatten To XML(6:w230) -> (2:w220:string)
            n110 = call "File Dialog2"("start path"=w224, "prompt"=w223, "pattern (all files)"=w222) -> ("selected path"=w226:path, "error out"=w231:errorcluster)  [unwired: 9 in, 2 out]
            n111 = Open/Create/Replace File(file path (use dialog)=w226, error in=w231, operation (0:open)=T6."replace or create") -> (refnum out=w228:refnum<file>, error out=w232:errorcluster)  [unwired: 3 in, 1 out]
            n112 = Write to Text File(file (use dialog)=w228, text=w220, error in=w232) -> (refnum out=w227:refnum<file>, error out=w233:errorcluster)  [unwired: 1 in, 1 out]
            n113 = Close File(refnum=w227, error in=w233) -> (path=w214:path, error out=w215:errorcluster)
            n114 = property class="Theme Config"(reference=w217, error in=w215, "data member access:theme path"=w214) -> (reference out=w216:refnum<class "Theme Config.lvclass">, error out=w213:errorcluster)
            n115 = local write "LabVIEW material theme"(w214) -> ()
            n116 = local write "Tab Control file"(enum32{"convert", "load"}."load" ("Tab Control file")) -> ()
            n117 = local write "File Interaction"(enum32{"convert--buton", "load--buton"}."load--buton" ("File Interaction")) -> ()
            n118 = call <vilib>:"Clear Errors.vi"("error in (no error)"=w213, "specific error code to clear (0: all)"=43) -> ("error out"=w212:errorcluster)  [unwired: 4 in, 1 out]
          }
        }
      }
      event "preview": Value Change {
        n119 = event-data() -> ()  [unwired: 1 in, 1 out]
        n120 = vi-ref "ui--test the theme.vi"() -> (w237:refnum<vi>)
        n121 = invoke class="VI" method="FP.Open"(reference=w237) -> ()  [unwired: 4 in, 5 out]
      }
      event Mouse Down {
        n122 = event-data() -> ("CtlRef"=w245:refnum<vi>, "Button"=w241:u16)  [unwired: 1 in]
        n123 = case shown="1" w241 {
          tunnel: w245 -> [_ w249]
          tunnel: w240 -> [w246 w252]
          tunnel: [w246 w251] -> w239
          frame 0, Default {
          }
          frame 1 {
            n124 = local read "Theme Mode"() -> (w250:u16)
            n125 = control-ref of="Tab Control"() -> (w248:refnum<vi>)
            n126 = control-ref of="This VI"() -> (w247:refnum<vi>)
            n127 = call "Replace Scheme Color.vi"("Theme Mode"=w250, "Colorbox ref in"=w249, "This VI"=w247, "TabControl in"=w248, "Material Theme in"=w252) -> ("Material Theme out"=w251:refnum<class "Material Theme.lvclass">)  [unwired: 6 in]
          }
        }
      }
      event "tabs": Value Change {
        n128 = event-data() -> ()  [unwired: 1 in, 1 out]
        n129 = Type Cast(type=T1."buttons" ("Tab Control"), x="tabs") -> (*(type *) &x=w256:T1)
        n130 = local write "Tab Control"(w256) -> ()
      }
      event "File Interaction": Value Change {
        n131 = event-data() -> ()  [unwired: 1 in, 1 out]
        n132 = Type Cast(type=enum32{"convert", "load"}."convert" ("Tab Control file"), x="File Interaction") -> (*(type *) &x=w265:enum32{"convert", "load"})
        n133 = local write "Tab Control file"(w265) -> ()
      }
      event "palette": Value Change {
        n134 = event-data() -> ()  [unwired: 1 in, 1 out]
        n135 = invoke class="VI (strict)" method="Abort VI"(reference=w269) -> (reference out=w268:refnum<vi>, error out=w267:errorcluster)  [unwired: 2 in, 1 out]
        n136 = Close Reference(reference=w268, error in (no error)=w267) -> (error out=w271:errorcluster)
        n137 = call <vilib>:"Clear Errors.vi"("error in (no error)"=w271) -> ("error out"=w270:errorcluster)  [unwired: 5 in, 1 out]
        n138 = local read "Theme Mode"() -> (w281:u16)
        n139 = vi-ref "TSC Material Theme.lvlib:Material-Scheme.lvclass:View-User Colors.vi"() -> (w276:refnum<vi>)
        n140 = call "Get Scheme.vi"("Theme"=w281, "Material Theme in"=w282) -> ("Material-Scheme"=w280:refnum<class "Material-Scheme.lvclass">)  [unwired: 7 in, 2 out]
        n141 = property class="VI Interface Type 0"(reference=w276, error in=w270) -> ("Name"=w279:string)  [unwired: 2 out]
        n142 = Open VI Reference(type specifier VI Refnum (for type only)=w276, vi path=w279, options=128) -> (vi reference=w277:refnum<vi>, error out=w275:errorcluster)  [unwired: 3 in]
        n143 = call-by-ref "Start Asynchronous Call"(reference=w277, error in=w275, "Material-Scheme.lvclass"=w280) -> (reference out=w274:refnum<vi>)  [unwired: 11 in, 1 out]
      }
    }
    n144 = call <vilib>:"Simple Error Handler.vi"("error in (no error)"=w78) -> ()  [unwired: 4 in, 5 out]
  }
  n145 = Unregister For Events(event registration refnum=w31) -> (error out=w5:errorcluster)  [unwired: 1 in]
  n146 = flat-sequence {
    tunnel: w37 -> [w291]
    tunnel: w33 -> [w290]
    tunnel: w12 -> [w285]
    tunnel: w5 -> [_]
    tunnel: w4 -> [w284]
    frame #0 {
      # "close references"
      n147 = invoke class="VI (strict)" method="Abort VI"(reference=w285) -> (reference out=w286:refnum<vi>, error out=w287:errorcluster)  [unwired: 2 in, 1 out]
      n148 = invoke class="VI" method="Abort VI"(reference=w284) -> (reference out=w289:refnum<vi>, error out=w288:errorcluster)  [unwired: 2 in, 1 out]
      n149 = control-ref of="This VI"() -> (w283:refnum<vi>)
      n150 = Close Reference(reference=w291) -> ()  [unwired: 1 in, 1 out]
      n151 = Close Reference(reference=w290) -> ()  [unwired: 1 in, 1 out]
      n152 = invoke class="VI" method="FP.Close"(reference=w283) -> ()  [unwired: 2 in, 3 out]
      n153 = Close Reference(reference=w286, error in (no error)=w287) -> ()  [unwired: 1 out]
      n154 = Close Reference(reference=w289, error in (no error)=w288) -> ()  [unwired: 1 out]
    }
  }
